vi "t1.vi"() -> ()   [LabVIEW 2020]
uses:
  <userlib>/KQD LabVIEW User/Serial/Controls/SERIAL PortConfig.ctl
  <userlib>/KQD LabVIEW User/Serial/Controls/SERIAL BaudRate.ctl
  <userlib>/Amira UART/Public/TypeDefs/AUART StepDir.ctl
  <userlib>/Amira UART/Amira UART.lvclass
  <userlib>/KQD LabVIEW User/Serial/Serial.lvlib
panel:
  in  "Folder":path
  in  "Strip":enum16{"Surface", "Blader"}(ring)
  out "FrontOpen":dbl
  out "BackOpen":dbl
  out "FrontClose":dbl
  out "BackClose":dbl
  in  "Start":cluster{"Steps":i32, "Rates":i32}={"Steps"=700, "Rates"=200}
  out "Position":dbl[](graph)
  in  "DAQ":tag="Dev1/port0"
  out "UART":string
  in  "ComPort":refnum<visa-resource-name>
  in  "Config":T1={"BaudRate"=enum."460800", "StopBits"=10, "DataBits"=8, "Parity"=enum."None", "FlowControl"=2, "TimeOut"=1000, "TermChar"=10, "ReadTermEn"=TRUE} {"TermChar" format="%.0x"; "FlowControl" items=["None", "XON/XOFF", "RTS/CTS", "XON/XOFF & RTS/CTS", "DTR/DSR", "XON/XOFF & DTR/DSR"]; "DataBits" min=5 max=8 step=1; "StopBits" items=["1.0"=10, "1.5"=15, "2.0"=20]}
  out "ErrOut":errorcluster
  in  "ErrIn":errorcluster
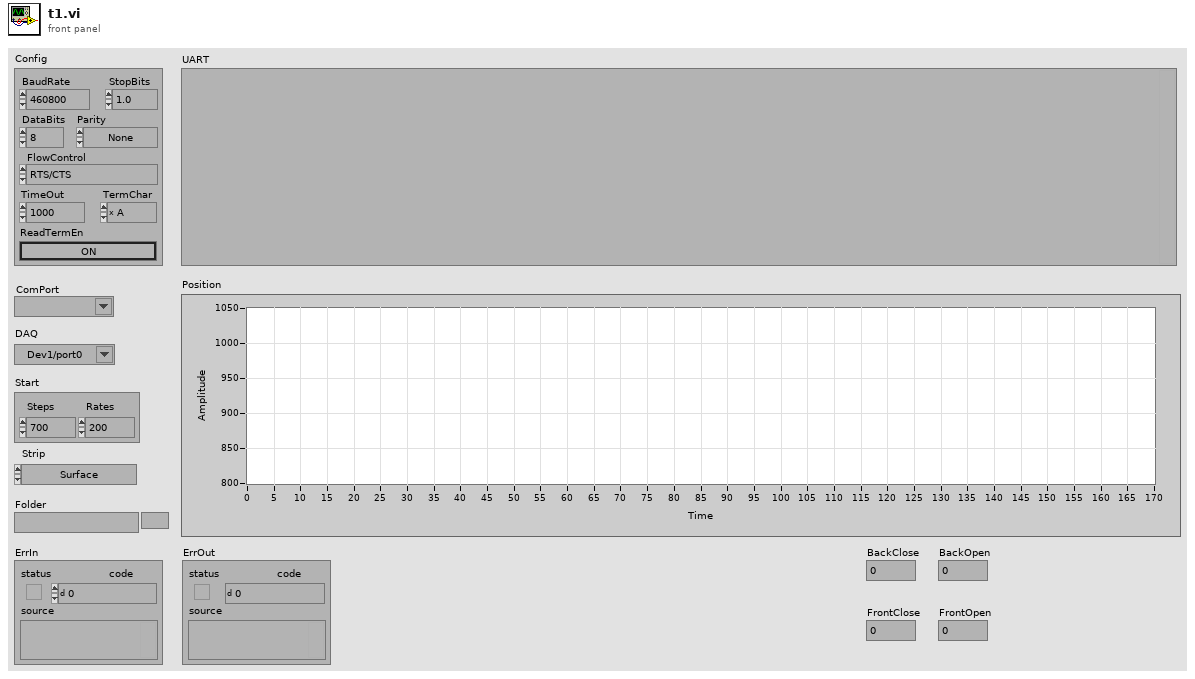
[diagram p1: front panel]
types:
  T1 = typedef "Serial.lvlib/SERIAL PortConfig.ctl" = cluster{"BaudRate":T2, "StopBits":u16, "DataBits":u16, "Parity":enum16{"None", "Odd", "Even", "Mark", "Space"}, "FlowControl":u16, "TimeOut":u32, "TermChar":u8, "ReadTermEn":bool}
  T2 = typedef "SERIAL BaudRate.ctl" = enum16{"2400", "4800", "7200", "9600", "14400", "19200", "28800", "38400", "57600", "115200", "128000", "230400", "460800", "921600"}
  T3 = typedef "Amira UART.lvclass/AUART StepDir.ctl" = enum16{"", "compress", "decompress"}
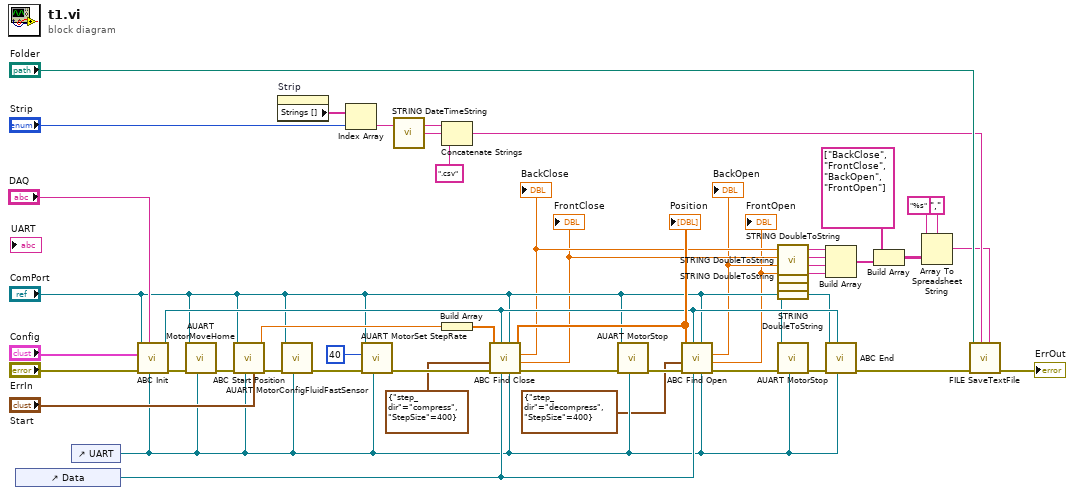
[diagram p0: block diagram]
diagram:
  n1 = control-ref of="Data"() -> (w28:refnum<vi>)
  n2 = control-ref of="UART"() -> (w25:refnum<vi>)
  n3 = call "ABC Init.vi"("UART"=w25, "DAQ"="DAQ", "ErrIn"="ErrIn", "PortConfig"="Config", "ComPort"="ComPort") -> ("ErrOut"=w41:errorcluster, "DaqTask"=w29:refnum<k21>)  [unwired: 5 in]
  n4 = call <userlib>:"AUART MotorMoveHome.vi"("UART"=w25, "ErrIn"=w41, "Port"="ComPort") -> ("ErrOut"=w39:errorcluster)  [unwired: 7 in, 1 out]
  n5 = call "ABC Start Position.vi"("Start"="Start", "UART"=w25, "ErrIn"=w39, "ComPort"="ComPort") -> ("ErrOut"=w38:errorcluster, "LastPos"=w35:dbl)  [unwired: 6 in]
  n6 = property on="Strip" class="Enum (strict)"() -> ("Strings []"=w17:string[])  [unwired: 2 in, 2 out]
  n7 = call <userlib>:"AUART MotorConfigFluidFastSensor.vi"("UART"=w25, "ErrIn"=w38, "Port"="ComPort") -> ("ErrOut"=w44:errorcluster)  [unwired: 8 in]
  n8 = Index Array(array=w17, index="Strip") -> (element=w15:string)
  n9 = call <userlib>:"AUART MotorSet StepRate.vi"("UART"=w25, "ErrIn"=w44, "step_rate"=40, "Port"="ComPort") -> ("ErrOut"=w42:errorcluster)  [unwired: 7 in]
  n10 = call <userlib>:"STRING DateTimeString.vi"() -> ("DateTimeStr"=w14:string)  [unwired: 2 in]
  n11 = Concatenate Strings(w15, w14, ".csv" ("string")) -> (w11:string)
  n12 = Build Array(w35) -> (w36:dbl[])
  n13 = call "ABC Find Close.vi"("UART"=w25, "ComPort"="ComPort", "Data"=w28, "DaqTask"=w29, "ErrIn"=w42, "DirSize"=cluster{"step_dir":T3, "StepSize":i32} {"step_dir"=enum."compress", "StepSize"=400}, "DataIn"=w36) -> ("ErrOut"=w33:errorcluster, "FrontClose"=w22:dbl, "BackClose"=w23:dbl, "DataOut"=w30:dbl[])  [unwired: 1 in]
  "Position" <- w30
  "BackClose" <- w23
  "FrontClose" <- w22
  n14 = call <userlib>:"AUART MotorStop.vi"("UART"=w25, "ErrIn"=w33, "Port"="ComPort") -> ("ErrOut"=w32:errorcluster)  [unwired: 8 in]
  n15 = call "ABC Find Open.vi"("UART"=w25, "ComPort"="ComPort", "Data"=w28, "DaqTask"=w29, "ErrIn"=w32, "DirSize"=cluster{"step_dir":T3, "StepSize":i32} {"step_dir"=enum."decompress", "StepSize"=400}, "DataIn"=w30) -> ("ErrOut"=w31:errorcluster, "FrontOpen"=w20:dbl, "BackOpen"=w21:dbl)  [unwired: 1 in, 1 out]
  "BackOpen" <- w21
  "FrontOpen" <- w20
  n16 = call <userlib>:"STRING DoubleToString.vi"("Num"=w23) -> ("DblStr"=w10:string)  [unwired: 3 in]
  n17 = call <userlib>:"STRING DoubleToString.vi"("Num"=w22) -> ("DblStr"=w9:string)  [unwired: 3 in]
  n18 = call <userlib>:"STRING DoubleToString.vi"("Num"=w21) -> ("DblStr"=w8:string)  [unwired: 3 in]
  n19 = call <userlib>:"STRING DoubleToString.vi"("Num"=w20) -> ("DblStr"=w7:string)  [unwired: 3 in]
  n20 = call <userlib>:"AUART MotorStop.vi"("UART"=w25, "ErrIn"=w31, "Port"="ComPort") -> ("ErrOut"=w26:errorcluster)  [unwired: 8 in]
  n21 = Build Array(w10, w9, w8, w7) -> (w5:string[])
  n22 = call "ABC End.vi"("UART"=w25, "DaqTask"=w29, "ErrIn"=w26, "ComPort"="ComPort") -> ("ErrOut"=w19:errorcluster)  [unwired: 7 in]
  n23 = Build Array(string[] ["BackClose", "FrontClose", "BackOpen", "FrontOpen"], w5) -> (w4:string[][])
  n24 = Array To Spreadsheet String(delimiter (Tab)=",", array=w4, 3:"%s" ("format string")) -> (spreadsheet string=w2:string)
  n25 = call <userlib>:"FILE SaveTextFile.vi"("Data"=w2, "File"=w11, "ErrIn"=w19, "Folder"="Folder") -> ("ErrOut"=→"ErrOut":errorcluster)  [unwired: 7 in]
